vi "uA_daq_change_shunt_resistors.vi"(8 "error in":errorcluster, 9 "Shunt Slector":enum16{"Shunt 3.333 Ohm", "Shunt 1 Ohm"}(ring), 11 "device name":tag="Dev4") -> (0 "error out":errorcluster)   [LabVIEW 2015]
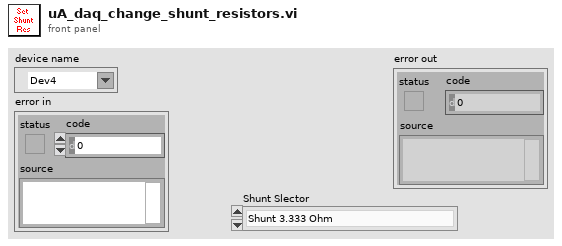
[diagram p1: front panel]
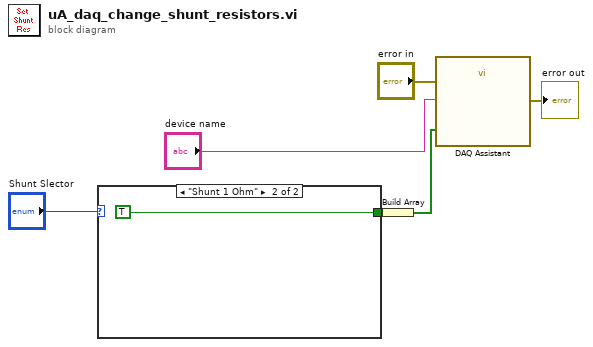
[diagram p0: block diagram]
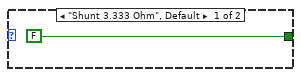
[diagram p2: hidden frame]
diagram:
  n1 = case shown="\"Shunt 1 Ohm\"" "Shunt Slector" {
    tunnel: [FALSE TRUE] -> w5
    frame "Shunt 3.333 Ohm", Default {
    }
    frame "Shunt 1 Ohm" {
    }
  }
  n2 = Build Array(w5) -> (w4:bool[])
  n3 = call "DAQ Assistant"("data"=w4, "error in"="error in", "device name"="device name") -> ("error out"=→"error out":errorcluster)  [unwired: 15 in, 1 out]
